vi "Stop Measurements.vi"(8 "error in (no error)":errorcluster, 11 "Measure Controller in":refnum<class "Process Controller.lvclass">) -> (0 "error out":errorcluster, 3 "Measure Controller out":refnum<class "Process Controller.lvclass">)   [LabVIEW 2016, in "Process Controller.lvclass"]
uses:
  Process Controller.lvclass
  C:/github/LabActor/Worker/Worker.lvclass
  C:/Program Files/National Instruments/LabVIEW 2016/vi.lib/ActorFramework/Actor/Actor.lvclass
  Worker/Worker.lvclass/Worker.ctl
  NHMFL_Core/Libraries/Instruments/Instrument Driver/Worker State.ctl
  Process Controller Messages/Stop Response Msg/Stop Response Msg.lvclass
  C:/github/LabActor/Template Module Messages/Self-Addressed Msg/Self-addressed Msg.lvclass
  Process Controller.lvclass/Process Controller.ctl
  <vilib>/ActorFramework/Actor/Actor.lvclass/Actor.ctl
  <vilib>/ActorFramework/Message Enqueuer/Message Enqueuer.lvclass/Message Enqueuer.ctl
  Template Module Messages/Self-Addressed Msg/Self-addressed Msg.lvclass/Self-addressed Msg.ctl
  Worker Messages/Stop Work Msg/Stop Work Msg.lvclass/Stop Work Msg.ctl
  Template Module/Write State.vi
  Read Active measurements enqueuers.vi
  Worker/Write Pause requested.vi
  Worker/Write Paused.vi
  Template Module Messages/Self-Addressed Msg/Write Return Enqueuer.vi
  Template Module/Read State.vi
  <vilib>/ActorFramework/Message Enqueuer/Init from Existing Queue.vi
  <vilib>/ActorFramework/Message Enqueuer/Enqueue.vi
  Worker Messages/Stop Work Msg/Stop Work Msg.lvclass
  C:/Program Files/National Instruments/LabVIEW 2016/vi.lib/ActorFramework/Message/Message.lvclass
  <vilib>/ActorFramework/Message Priority Queue/Priority Enqueue.vi
  <vilib>/ActorFramework/Message Enqueuer/Message Enqueuer.lvclass
  <vilib>/ActorFramework/Actor/Actor.lvclass
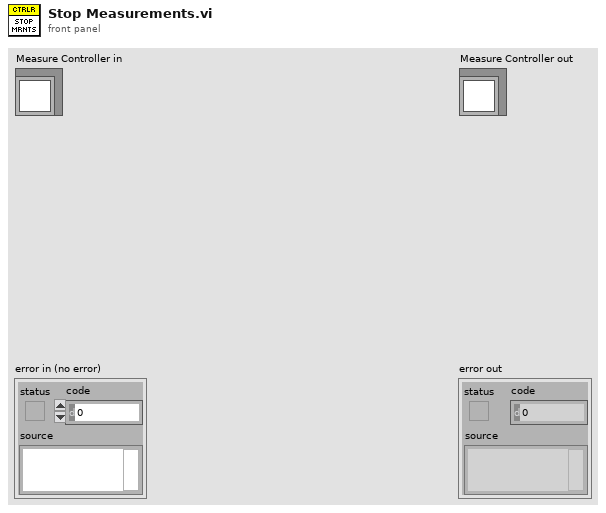
[diagram p1: front panel]
types:
  T1 = typedef "Worker State.ctl" = enum16{"Idle", "Starting", "Working", "Stopping"}
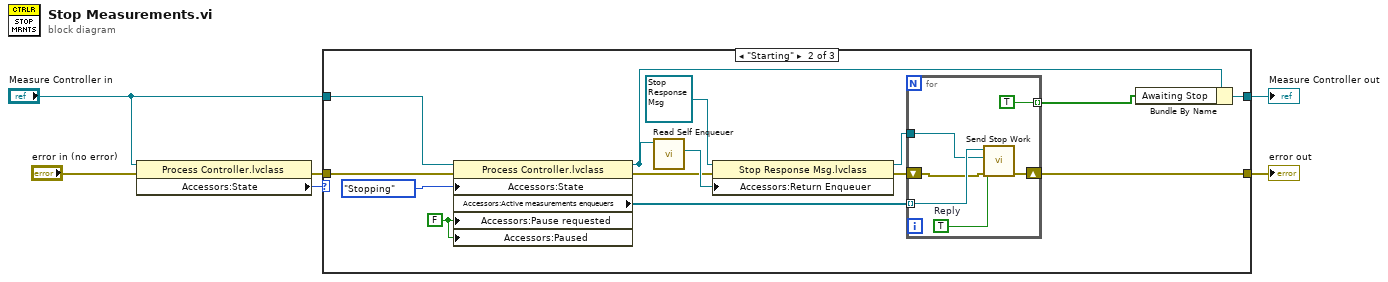
[diagram p0: block diagram]
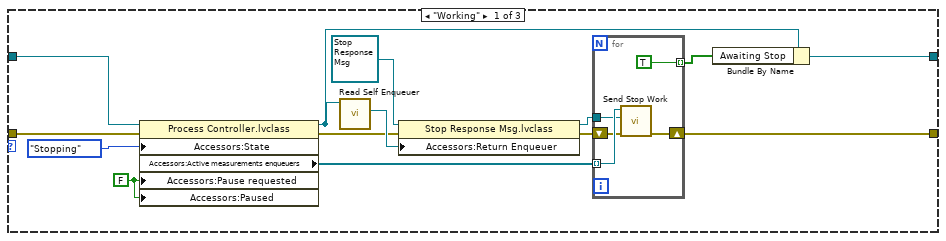
[diagram p2: hidden frame]
diagram:
  n1 = property class="Process Controller.lvclass"(reference="Measure Controller in", error in="error in (no error)") -> (error out=w1:errorcluster, "Accessors:State"=w2:T1)  [unwired: 1 out]
  n2 = case shown="\"Starting\"" w2 {
    tunnel: [w19 w38 w46] -> w6
    tunnel: [w9 w28 w47] -> w5
    tunnel: "Measure Controller in" -> [w20 w39 w47]
    tunnel: w1 -> [w10 w29 w46]
    frame "Working" {
      w7 = FALSE ("Pause requested")
      n3 = property class="Process Controller.lvclass"(reference=w20, error in=w10, "Accessors:State"=Worker_State."Stopping" ("State"), "Accessors:Pause requested"=w7, "Accessors:Paused"=w7) -> (reference out=w16:refnum<class "Process Controller.lvclass">, error out=w13:errorcluster, "Accessors:Active measurements enqueuers"=w18:refnum<class "Message Enqueuer.lvclass">[])
      n4 = call <vilib>:"Read Self Enqueuer.vi"("Actor"=w16) -> ("Self Enqueuer"=w14:refnum<class "Message Enqueuer.lvclass">)  [unwired: 10 in]
      n5 = property class="Stop Response Msg.lvclass"(reference=refnum<class "Stop Response Msg.lvclass"> refnum ("Stop Response Msg.lvclass"), error in=w13, "Accessors:Return Enqueuer"=w14) -> (reference out=w12:refnum<class "Stop Response Msg.lvclass">, error out=w11:errorcluster)
      n6 = for {
        tunnel: w18 -> [w25] mode=indexing
        shift-right: [w23] -> w19
        shift-left: w11 -> [w24]
        tunnel: w12 -> [w22]
        tunnel: [TRUE] -> w8 mode=indexing
        n7 = call "Send Stop Work.vi"("error in (no error)"=w24, "Reply to"=w22, "Message Enqueuer"=w25) -> ("error out"=w23:errorcluster)  [unwired: 7 in, 1 out]
      }
      n8 = Bundle By Name(cluster=w16, "Awaiting Stop"=w8) -> (w9:refnum<class "Process Controller.lvclass">)
    }
    frame "Starting" {
      w26 = FALSE ("Pause requested")
      n9 = property class="Process Controller.lvclass"(reference=w39, error in=w29, "Accessors:State"=Worker_State."Stopping" ("State"), "Accessors:Pause requested"=w26, "Accessors:Paused"=w26) -> (reference out=w35:refnum<class "Process Controller.lvclass">, error out=w32:errorcluster, "Accessors:Active measurements enqueuers"=w37:refnum<class "Message Enqueuer.lvclass">[])
      n10 = call <vilib>:"Read Self Enqueuer.vi"("Actor"=w35) -> ("Self Enqueuer"=w33:refnum<class "Message Enqueuer.lvclass">)  [unwired: 10 in]
      n11 = property class="Stop Response Msg.lvclass"(reference=refnum<class "Stop Response Msg.lvclass"> refnum ("Stop Response Msg.lvclass"), error in=w32, "Accessors:Return Enqueuer"=w33) -> (reference out=w31:refnum<class "Stop Response Msg.lvclass">, error out=w30:errorcluster)
      n12 = for {
        tunnel: w37 -> [w45] mode=indexing
        shift-right: [w43] -> w38
        shift-left: w30 -> [w44]
        tunnel: w31 -> [w42]
        tunnel: [TRUE] -> w27 mode=indexing
        w40 = TRUE  # Reply
        n13 = call "Send Stop Work.vi"("error in (no error)"=w44, "Reply"=w40, "Reply to"=w42, "Message Enqueuer"=w45) -> ("error out"=w43:errorcluster)  [unwired: 6 in, 1 out]
      }
      n14 = Bundle By Name(cluster=w35, "Awaiting Stop"=w27) -> (w28:refnum<class "Process Controller.lvclass">)
    }
    frame "Idle", Default {
    }
  }
  "error out" <- w6
  "Measure Controller out" <- w5
